vi "Interface_Dispatch_Initialize Module.vi"(8 "error in (no error)":errorcluster, 11 "Dispatch_SOC Control in":refnum<class "Dispatch_SOC Control.lvclass">) -> (0 "error out":errorcluster, 2 "TagDescriptions":refnum<class "tag descriptor.lvclass">[](array[class]), 3 "Dispatch_SOC Control out":refnum<class "Dispatch_SOC Control.lvclass">)   [LabVIEW 2015, in "Dispatch_SOC Control.lvclass"]
uses:
  Dispatch_SOC Control.lvclass
  <vilib>/NI/Tag Bus/tag/tag descriptor.lvclass
  TagBus/TagBus.lvclass
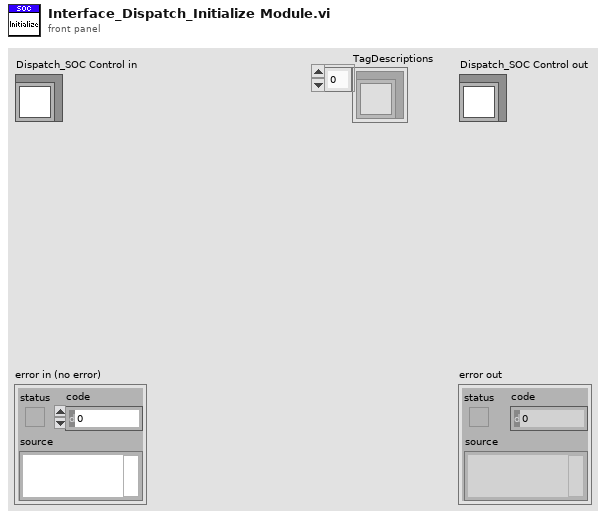
[diagram p1: front panel]
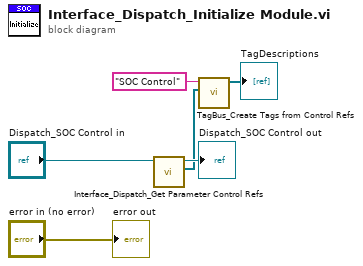
[diagram p0: block diagram]
diagram:
  n1 = call-dynamic "Interface_Dispatch_Get Parameter Control Refs.vi"("Dispatch_SOC Control in"="Dispatch_SOC Control in") -> ("Controls[]"=w3:refnum<vi>[], "Dispatch_SOC Control out"=→"Dispatch_SOC Control out":refnum<class "Dispatch_SOC Control.lvclass">)  [unwired: 8 in, 1 out]
  n2 = call "TagBus_Create Tags from Control Refs.vi"("Array"=w3, "Process Name"="SOC Control") -> ("TagDescriptions"=→"TagDescriptions":refnum<class "tag descriptor.lvclass">[])  [unwired: 9 in]
  "error out" <- "error in (no error)"
